vi "Abort Generation.vi"(0 "RFSG handle":refnum<k15>, 5 "Timeout (ms)":dbl=1000.0 format="%#_6p", 11 "error in (no error)":errorcluster) -> (4 "RFSG handle out":refnum<k15>, 15 "error out":errorcluster)   [LabVIEW 2019, in "SG.lvlib"]
doc: "Notifies running scripts configured with <b>Configure Continuous Generation</b> or <b>Configure Bursted Generation</b> to enter the cleanup state, and then aborts generation. This function ensures that these scripts always reach a finished state before aborting, so as to ensure the DUT is in the desired state at the end of generation."
uses:
  SG.lvlib
  <instrlib>/niRFSG/niRFSG.llb/niRFSG Script Trigger IDs.ctl
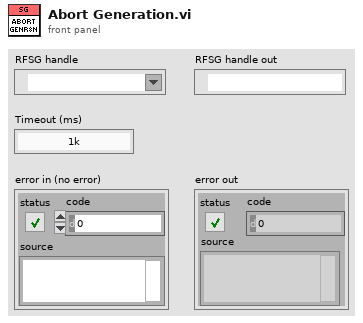
[diagram p1: front panel]
types:
  T1 = typedef "niRFSG Script Trigger IDs.ctl" = string
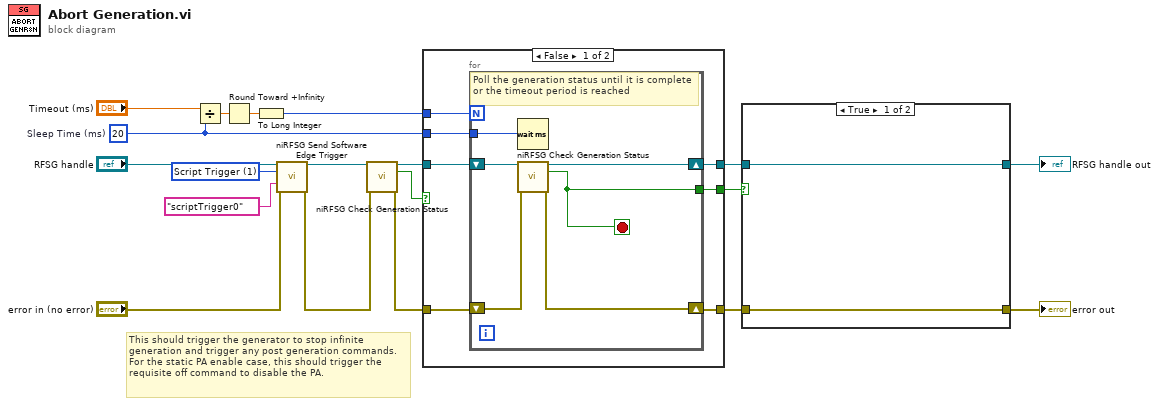
[diagram p0: block diagram]
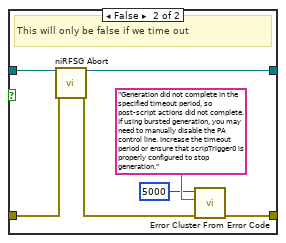
[diagram p2: hidden frame]
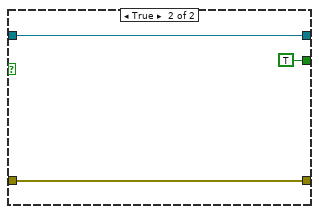
[diagram p3: hidden frame]
diagram:
  w1 = u32 20  # Sleep Time (ms)
  w17 = 1 items=["Start Trigger", "Script Trigger"] ("trigger type")
  # "This should trigger the generator to stop infinite generation and trigger any post generation commands. For the static PA enable case, this should trigger the requisite off command to disable the PA."
  n1 = Divide(x="Timeout (ms)", y=w1) -> (x/y=w13:dbl)
  n2 = Round Toward +Infinity(x=w13) -> (ceil(x): smallest int >= x=w7:dbl)
  n3 = To Long Integer(number=w7) -> (32bit integer=w6:i32)
  n4 = call <instrlib>:"niRFSG Send Software Edge Trigger.vi"("instrument handle"="RFSG handle", "trigger type"=w17, "trigger ID"=T1 "scriptTrigger0", "error in"="error in (no error)") -> ("instrument handle out"=w18:refnum<k15>, "error out"=w12:errorcluster)  [unwired: 10 in]
  n5 = call <instrlib>:"niRFSG Check Generation Status.vi"("instrument handle"=w18, "error in"=w12) -> ("instrument handle out"=w11:refnum<k15>, "done?"=w8:bool, "error out"=w9:errorcluster)  [unwired: 11 in]
  n6 = case shown="False" w8 {
    tunnel: w11 -> [w26 w35]
    tunnel: [w25 w35] -> w10
    tunnel: w9 -> [w24 w34]
    tunnel: [w23 w34] -> w4
    tunnel: w6 -> [w22 _]
    tunnel: [w21 TRUE ("done?")] -> w2
    tunnel: w1 -> [w20 _]
    frame False {
      n7 = for {
        N: w22 -> [_]
        shift-right: [w31] -> w25
        shift-left: w26 -> [w32]
        shift-right: [w29] -> w23
        shift-left: w24 -> [w30]
        tunnel: [w28] -> w21
        tunnel: w20 -> [w27]
        stop <- w28 stop-if-true
        # "Poll the generation status until it is complete or the timeout period is reached"
        n8 = Wait (ms)(milliseconds to wait=w27) -> ()  [unwired: 1 out]
        n9 = call <instrlib>:"niRFSG Check Generation Status.vi"("instrument handle"=w32, "error in"=w30) -> ("instrument handle out"=w31:refnum<k15>, "done?"=w28:bool, "error out"=w29:errorcluster)  [unwired: 11 in]
      }
    }
    frame True {
    }
  }
  n10 = case shown="True" w2 {
    tunnel: w10 -> [w37 w43]
    tunnel: [w37 w42] -> w5
    tunnel: w4 -> [w36 w41]
    tunnel: [w36 w39] -> w3
    frame True {
    }
    frame False {
      # "This will only be false if we time out"
      n11 = call <instrlib>:"niRFSG Abort.vi"("instrument handle"=w43, "error in"=w41) -> ("instrument handle out"=w42:refnum<k15>, "error out"=w40:errorcluster)  [unwired: 12 in]
      n12 = call <vilib>:"Error Cluster From Error Code.vi"("error in (no error)"=w40, "error message (\"\")"="Generation did not complete in the specified timeout period, so post-script actions did not complete. If using bursted generation, you may need to manually disable the PA control line. Increase the timeout period or ensure that scripTrigger0 is properly configured to stop generation.", "error code (0)"=5000) -> ("error out"=w39:errorcluster)  [unwired: 6 in]
    }
  }
  "RFSG handle out" <- w5
  "error out" <- w3
